vi "Write Configuration.vi"(8 "error in (no error)":errorcluster, 10 "Configuration":variant, 11 "JSON Config File in":refnum<class "JSON Config File.lvclass">) -> (0 "error out":errorcluster, 3 "JSON Config File out":refnum<class "JSON Config File.lvclass">)   [LabVIEW 2019, in "JSON Config File.lvclass"]
doc: "JKI JSON 1.1.10.37\nTomi Maila - JKI\nCopyright (c) 2017, JKI"
uses:
  JSON Config File.lvclass
  JSON Config File.lvclass/JSON Config File.ctl
  vi.lib/addons/_JKI.lib/Serialization/JSON/JKI JSON Serialization.lvlib
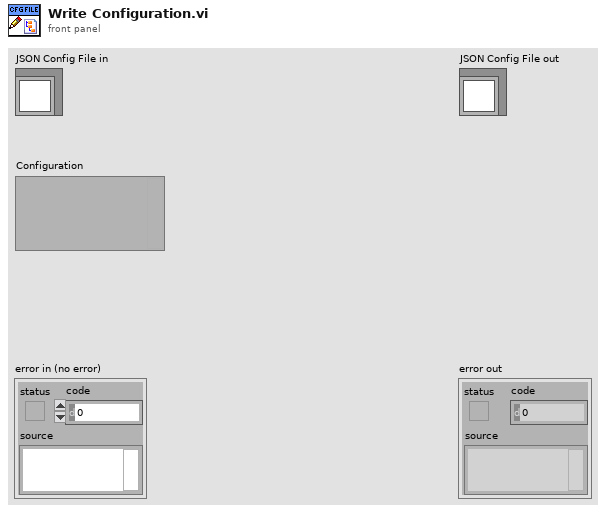
[diagram p1: front panel]
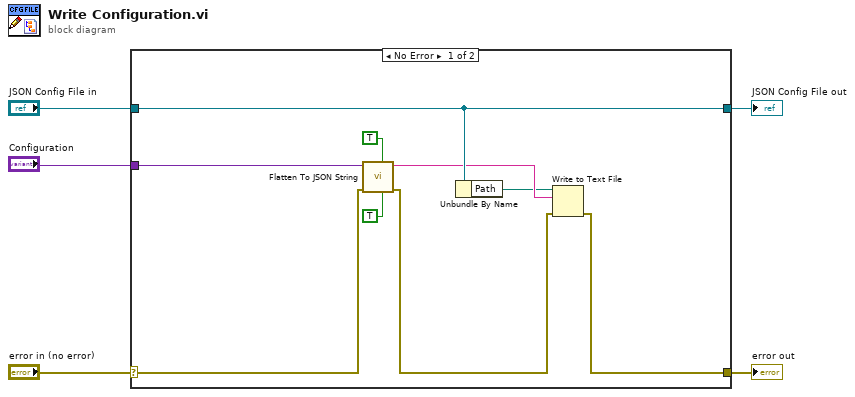
[diagram p0: block diagram]
diagram:
  n1 = case shown="No Error" "error in (no error)" {
    selector: "error in (no error)" -> [w12 w16]
    tunnel: [w7 w16] -> w4
    tunnel: [w14 w15] -> w2
    tunnel: "JSON Config File in" -> [w14 w15]
    tunnel: "Configuration" -> [w13 _]
    frame No Error {
      n2 = call "Flatten To JSON String.vi"("Enums As String (F)"=TRUE ("Nulls as Defaults (F)"), "Numeric Extensions (F)"=TRUE, "error in (no error)"=w12, "Variant"=w13) -> ("error out"=w6:errorcluster, "JSON String"=w9:string)  [unwired: 6 in]
      n3 = Unbundle By Name(w14) -> ("Path"=w8:path)
      n4 = Write to Text File(file (use dialog)=w8, text=w9, error in=w6) -> (error out=w7:errorcluster)  [unwired: 1 in, 2 out]
    }
    frame Error {
    }
  }
  "error out" <- w4
  "JSON Config File out" <- w2
